vi "Read Buffer Count.vi"(8 "error in":errorcluster, 11 "VISA resource name":refnum<visa-resource-name>) -> (0 "error out":errorcluster, 1 "Confirmation Response":string, 2 "count":i32, 3 "VISA resource name out":refnum<visa-resource-name>)   [LabVIEW 2024, in "Micron Optics sm130.lvlib"]
uses:
  Micron Optics sm130.lvlib
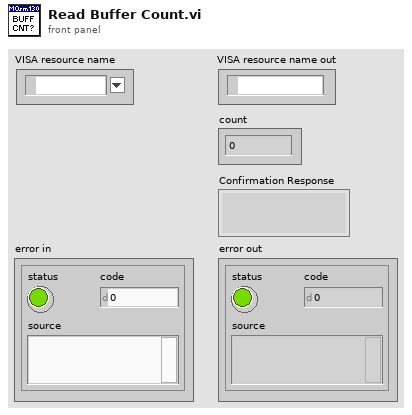
[diagram p1: front panel]
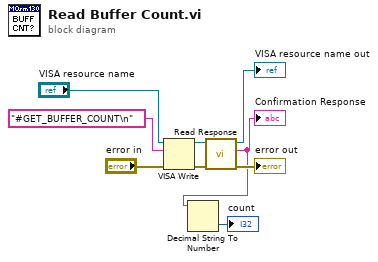
[diagram p0: block diagram]
diagram:
  n1 = VISA Write(VISA resource name="VISA resource name", write buffer="#GET_BUFFER_COUNT\n" ("string"), error in (no error)="error in") -> (VISA resource name out=w6:refnum<visa-resource-name>, error out=w5:errorcluster)  [unwired: 1 out]
  n2 = call "Read Response.vi"("error in (no error)"=w5, "VISA resource name"=w6) -> ("error out"=→"error out":errorcluster, "Confirmation Response"=w2:string, "VISA resource name out"=→"VISA resource name out":refnum<visa-resource-name>)  [unwired: 7 in]
  "Confirmation Response" <- w2
  n3 = Decimal String To Number(string=w2) -> (number=→"count":i32)  [unwired: 2 in, 1 out]
